vi "input.vi"(8 "error in":errorcluster, 10 "data table in":T1, 11 "TEC runtime in":refnum<class "TEC runtime.lvclass">) -> (0 "error out":errorcluster, 2 "data table out":T1, 3 "TEC runtime out":refnum<class "TEC runtime.lvclass">)   [LabVIEW 2013, in "TEC runtime.lvclass"]
doc: "Provides an interface for reading data from a module at runtime. While this interface performs no operations, a child should provide an override which may read from any open sessions, references, or interfaces."
uses:
  TEC runtime.lvclass
  <vilib>/NI/Tag Bus/table/data table.ctl
  TEC runtime.lvclass/TEC runtime.ctl
  <vilib>/NI/Tag Bus/table/data table.lvlib
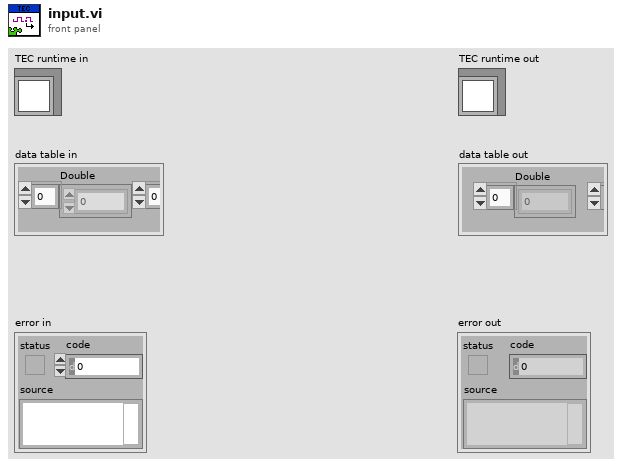
[diagram p1: front panel]
types:
  T1 = typedef "tag bus.lvlib/data table.lvlib/data table.ctl" = cluster{"Double":dbl[], "Single":sgl[], "I64":i64[], "I32":i32[], "I16":i16[], "I8":i8[], "U64":u64[], "U32":u32[], "U16":u16[], "U8":u8[], "Boolean":bool[], "String":string[], "Array of Double":cluster{"DBL Array":dbl[]}[], "Array of Single":cluster{"SGL Array":sgl[]}[], "Array of I64":cluster{"I64 Array":i64[]}[], "Array of I32":cluster{"I32 Array":i32[]}[], "Array of I16":cluster{"I16 Array":i16[]}[], "Array of I8":cluster{"I8 Array":i8[]}[], "Array of U64":cluster{"U64 Array":u64[]}[], "Array of U32":cluster{"U32 Array":u32[]}[], "Array of U16":cluster{"U16 Array":u16[]}[], "Array of U8":cluster{"U8 Array":u8[]}[], "Array of Boolean":cluster{"Boolean Array":bool[]}[], "Array of String":cluster{"String Array":string[]}[]}
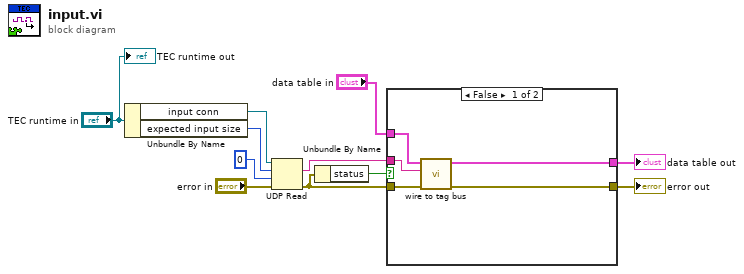
[diagram p0: block diagram]
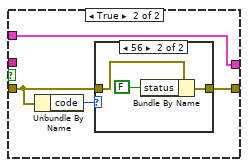
[diagram p2: hidden frame]
diagram:
  n1 = Unbundle By Name("TEC runtime in") -> ("input conn"=w10:refnum<k16>, "expected input size"=w9:i32)
  n2 = UDP Read(connection ID=w10, max size (548)=w9, timeout ms (25000)=0, 8:"error in") -> (data out=w3:string, error out=w1:errorcluster)  [unwired: 3 out]
  n3 = Unbundle By Name(w1) -> ("status"=w2:bool)
  n4 = case shown="False" w2 {
    tunnel: "data table in" -> [w14 w17]
    tunnel: [w16 w18] -> w5
    tunnel: [w15 w17] -> w4
    tunnel: w3 -> [w13 _]
    tunnel: w1 -> [w12 w19]
    frame False {
      n5 = call "wire to tag bus.vi"("error in"=w12, "wire data"=w13, "data table in"=w14) -> ("error out"=w16:errorcluster, "data table out"=w15:T1)  [unwired: 7 in]
    }
    frame True {
      n6 = Unbundle By Name(w19) -> ("code"=w20:i32)
      n7 = case shown="56" w20 {
        tunnel: w19 -> [w21 w24]
        tunnel: [w21 w22] -> w18
        frame Default {
        }
        frame 56 {
          n8 = Bundle By Name(cluster=w24, "status"=FALSE) -> (w22:errorcluster)
        }
      }
    }
  }
  "error out" <- w5
  "data table out" <- w4
  "TEC runtime out" <- "TEC runtime in"
